vi "LIDAR Data Loop.vi"() -> ()   [LabVIEW 2017]
uses:
  <vilib>/Platform/TimedLoop/XDataNode/timing_clust.ctl
  <vilib>/Platform/TimedLoop/XDataNode/nitl_modes.ctl
  <vilib>/Platform/TimedLoop/XDataNode/wakeup.ctl
  <vilib>/Platform/TimedLoop/XDataNode/XDataNode.xnode
  <vilib>/Platform/TimedLoop/XDataNode/XDNodeRunTimeDep.lvlib
panel:
  in  "filter?":bool=TRUE
  in  "median window size":i32=5
  in  "end point (120°)":dbl=100.0
  in  "start point (-120°)":dbl=-100.0
  out "error out":errorcluster
  in  "stop?":bool
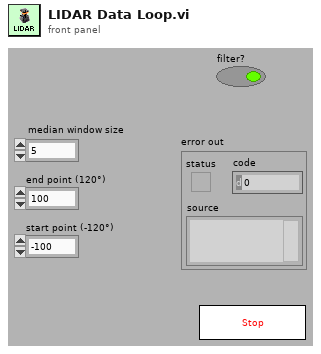
[diagram p1: front panel]
types:
  T1 = typedef "XDNodeRunTimeDep.lvlib/timing_clust.ctl" = cluster{"Expected End [f-1]":u64, "Actual End [f-1]":u64, "Finished Late? [f-1]":bool, "Expected End [i-1]":u64, "Actual End [i-1]":u64, "Finished Late? [i-1]":bool, "Expected Start [i]":u64, "Actual Start [i]":u64, "Expected Start [f]":u64, "Actual Start [f]":u64, "Source Name":string, "Structure Name":string, "Period":i64, "Deadline":i64, "Offset":i64, "Start":i64, "Priority":i32, "Timeout":i32, "Mode":T2, "Wakeup Reason":T3, "Error":errorcluster, "Source Type":string, "Secondary Source Type":string, "Global End Time":u64, "Global Start Time":u64, "Frame Duration":u64, "Iteration Duration":u64, "Assigned CPU":i32, "I/O Scan Engine Mode":u32}
  T2 = typedef "XDNodeRunTimeDep.lvlib/nitl_modes.ctl" = enum32{"No Change", "Process missed periods, maintain original phase", "Discard missed periods, maintain original phase", "Process missed periods, ignore original phase", "Discard missed periods, ignore original phase"}
  T3 = typedef "XDNodeRunTimeDep.lvlib/wakeup.ctl" = enum32{"Normal", "Aborted", "Asynchronous wakeup", "Timing source error", "Timed loop error", "Timeout"}
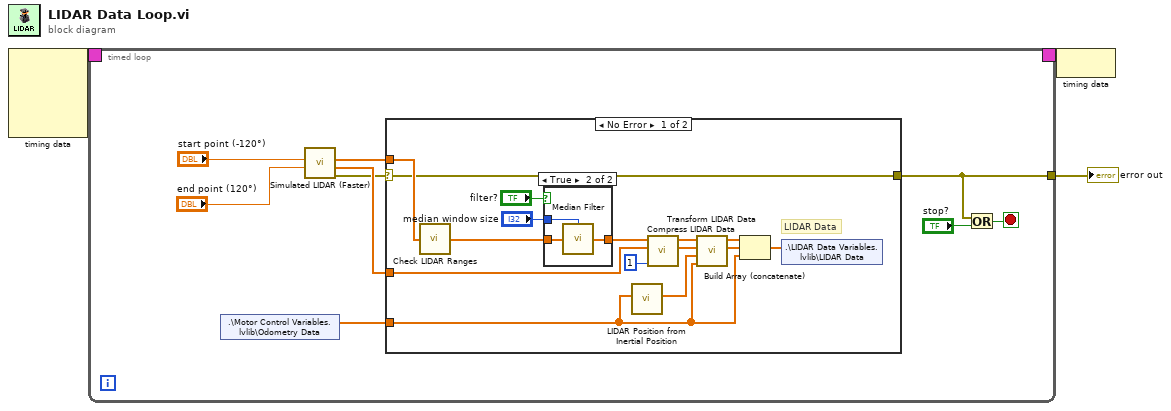
[diagram p0: block diagram]
diagram:
  n1 = node-c288() -> (w3:T1)  [unwired: 4 out]
  n2 = timed-loop {
    timing: w3 -> [_]
    timing-out: [_] -> w2
    tunnel: [w4] -> w1
    stop <- w6 stop-if-true
    n3 = shared-variable ".\\Motor Control Variables.lvlib\\Odometry Data"() -> (w10:dbl[])  [unwired: 1 in, 1 out]
    n4 = call "Simulated LIDAR (Faster).vi"("End Point (120°)"="end point (120°)", "Start Point (-120°)"="start point (-120°)") -> ("error out"=w5:errorcluster, "Direction"=w11:dbl[], "Magnitude"=w12:dbl[])  [unwired: 7 in]
    n5 = case shown="No Error" w5 {
      selector: w5 -> [w13 w32]
      tunnel: w12 -> [w24 _]
      tunnel: w11 -> [w26 _]
      tunnel: w10 -> [w14 _]
      tunnel: [w13 w32] -> w4
      frame No Error {
        # "LIDAR Data"
        n6 = call "Check LIDAR Ranges.vi"("Magnitude"=w24) -> ("Magnitude out"=w23:dbl[])  [unwired: 4 in]
        n7 = case shown="True" "filter?" {
          tunnel: w23 -> [w28 w31]
          tunnel: [w28 w30] -> w22
          tunnel: "median window size" -> [_ w29]
          frame False {
          }
          frame True {
            n8 = call "Median Filter.vi"("Values"=w31, "Median Window Size"=w29) -> ("Filtered Values"=w30:dbl[])
          }
        }
        n9 = call "LIDAR Position from Inertial Position.vi"("CM X, Y, Theta"=w14) -> ("LIDAR X, Y, Theta"=w17:dbl[])  [unwired: 10 in]
        n10 = call "Compress LIDAR Data.vi"("Compression Factor"=1 ("compress"), "Direction"=w26, "Magnitude"=w22) -> ("Compressed Direction"=w18:dbl[], "Compressed Magnitude"=w19:dbl[])  [unwired: 7 in]
        n11 = call "Transform LIDAR Data.vi"("New Orientation (X m, Y m, T rad)"=w14, "Orientation (X m, Y m, T rad)"=w17, "Direction (deg)"=w18, "Magnitude (mm)"=w19) -> ("Direction out (rad)"=w15:dbl[], "Magnitude out (m)"=w16:dbl[])  [unwired: 5 in, 1 out]
        n12 = Build Array (concatenate)(w16, w15, w14) -> (w27:dbl[])
        n13 = shared-variable ".\\LIDAR Data Variables.lvlib\\LIDAR Data"(w27) -> ()  [unwired: 1 in, 1 out]
      }
      frame Error {
      }
    }
    n14 = Or(x=w4, y="stop?") -> (x .or. y?=w6:bool)
  }
  "error out" <- w1
  n15 = node-c288(w2) -> ()
